vi "Keithley_IV Sweep.vi"() -> ()   [LabVIEW 2023]
uses:
  <instrlib>/Keithley 24XX/Public/Data/Read (Multiple Points).vi
  <vilib>/Utility/file.llb/Write Delimited Spreadsheet (DBL).vi
  <instrlib>/Keithley 24XX/Keithley 24XX.lvlib
  <vilib>/Analysis/NI_AALBase.lvlib
panel:
  in  "Current Range":i32(ring)=9 items=["mA"=3, "uA"=6, "nA"=9, "pA"=12]
  in  "path1 (folder + filename)":string="C:\\Users\\Carter Fox\\Documents\\probe data\\haolin\\"
  in  "Clear Plot":bool
  out "V-R":cluster{dbl[], dbl[]}(graph)={array[210 elements], [-5206154.0, -5436176.5, -5739949.7, -5522194.0, -5591894.0, -5776459.2, -5867751.5, -6153851.6, -6313039.5, -6546061.5, -6597968.0, -6737600.2, -6698442.5, -7003709.2, -7214062.5, -7227454.5, -7272324.7, -7315603.9, -8180765.4, -8370442.8, -8414466.4, -8558549.3, -8623235.6, -8485305.5, -8755154.4, -8913668.4, -8903585.8, -9356989.8, -9704273.0, -9888072.0, -9952694.2, -9462271.8, -9546720.8, -9151506.4, -9245727.0, -9130111.6, -8978078.6, -8980554.6, -8489626.5, -8766153.2, -8319403.2, -8056017.5, -8056376.9, -8148951.2, -8290770.6, -8061892.8, -8432694.3, -7918641.3, -7639503.0, -7371750.2, -7094581.9, -7089260.7, -6911397.3, -6586929.4, -6559722.9, -6559116.8, -6675187.5, -6447627.2, -6482316.2, -6441410.0, -6243156.7, -6007642.8, -5846703.5, -5641418.7, -5340011.0, -5222064.5, -5127084.4, -4771776.9, -4726834.2, -4488893.0, -4468031.1, -4344945.0, -4048716.15, -3995032.65, -3752934.4, -3515571.6, -3463041.0, -3307454.35, -3134452.0, -2865820.95, -2547093.35, -2451008.65, -2457232.75, -2264473.6, -2175654.9, -2075257.2, -1909759.55, -1690629.675, -1579277.55, -1439608.375, -1373833.05, -1280688.85, -1160609.625, -1028561.1, -853697.775, -738975.9375, -562712.525, -421306.975, -280443.56875, -143034.9875, 63.17793960571289, 142192.96875, 291373.54375, 450531.90625, 621629.55, 768361.2125, 936739.7125, 1078183.425, 1179651.7, 1308632.225, 1450103.325, 1578941.4, 1695594.975, 1815470.625, 2031218.15, 2205003.75, 2328910.65, 2527442.05, 2713821.7, 2773816.05, 2956326.5, 3094152.75, 3352913.7, 3405746.95, 3650903.3, 3816338.6, 3902421.4, 4254766.2, 4020501.7, 4199413.25, 4104189.3, 4316808.8, 4500217.9, 4625444.2, 4743101.6, 4847240.1, 4922873.9, 4963421.7, 5222360.7, 5435161.8, 5710479.7, 5953065.3, 5751540.2, 6185232.5, 6362707.2, 6258723.7, 6472245.0, 6749964.3, 6819459.9, 7089945.2, 7093988.2, 7265070.4, 7419388.4, 7450760.6, 7840890.3, 8010362.7, 8154184.9, 8595993.2, 8615776.8, 8657309.2, 8661124.2, 9076304.6, 8945453.0, 8963302.6, 9164656.4, 8956432.8, 9417630.4, 9845593.0, 9819956.8, 9964719.4, 9728544.4, 9516818.0, 9817531.6, 9995574.4, 9686989.6, 9619119.0, 9093431.0, 9016631.4, 9295223.0, 9272582.4, 9244173.2, 9498271.4, 8724864.2, 8299565.0, 8137673.6, 8124835.6, 8086662.6, 8106061.7, 7453452.1, 7138170.5, 6848874.7, 6885388.3, 6666333.2, 6471642.2, 6353635.0, 5981459.0, 5628015.5, 5593445.0, 5523823.4, 5316410.3, 5433694.8, 5403524.7, 5133651.1, 4923655.6, 4705024.7, 4949501.6, 4856533.7, 4489112.1, 4293774.4, 4293774.4]}
  out "I-R":cluster{dbl[], dbl[]}(graph)={array[210 elements], [-5206154.0, -5436176.5, -5739949.7, -5522194.0, -5591894.0, -5776459.2, -5867751.5, -6153851.6, -6313039.5, -6546061.5, -6597968.0, -6737600.2, -6698442.5, -7003709.2, -7214062.5, -7227454.5, -7272324.7, -7315603.9, -8180765.4, -8370442.8, -8414466.4, -8558549.3, -8623235.6, -8485305.5, -8755154.4, -8913668.4, -8903585.8, -9356989.8, -9704273.0, -9888072.0, -9952694.2, -9462271.8, -9546720.8, -9151506.4, -9245727.0, -9130111.6, -8978078.6, -8980554.6, -8489626.5, -8766153.2, -8319403.2, -8056017.5, -8056376.9, -8148951.2, -8290770.6, -8061892.8, -8432694.3, -7918641.3, -7639503.0, -7371750.2, -7094581.9, -7089260.7, -6911397.3, -6586929.4, -6559722.9, -6559116.8, -6675187.5, -6447627.2, -6482316.2, -6441410.0, -6243156.7, -6007642.8, -5846703.5, -5641418.7, -5340011.0, -5222064.5, -5127084.4, -4771776.9, -4726834.2, -4488893.0, -4468031.1, -4344945.0, -4048716.15, -3995032.65, -3752934.4, -3515571.6, -3463041.0, -3307454.35, -3134452.0, -2865820.95, -2547093.35, -2451008.65, -2457232.75, -2264473.6, -2175654.9, -2075257.2, -1909759.55, -1690629.675, -1579277.55, -1439608.375, -1373833.05, -1280688.85, -1160609.625, -1028561.1, -853697.775, -738975.9375, -562712.525, -421306.975, -280443.56875, -143034.9875, 63.17793960571289, 142192.96875, 291373.54375, 450531.90625, 621629.55, 768361.2125, 936739.7125, 1078183.425, 1179651.7, 1308632.225, 1450103.325, 1578941.4, 1695594.975, 1815470.625, 2031218.15, 2205003.75, 2328910.65, 2527442.05, 2713821.7, 2773816.05, 2956326.5, 3094152.75, 3352913.7, 3405746.95, 3650903.3, 3816338.6, 3902421.4, 4254766.2, 4020501.7, 4199413.25, 4104189.3, 4316808.8, 4500217.9, 4625444.2, 4743101.6, 4847240.1, 4922873.9, 4963421.7, 5222360.7, 5435161.8, 5710479.7, 5953065.3, 5751540.2, 6185232.5, 6362707.2, 6258723.7, 6472245.0, 6749964.3, 6819459.9, 7089945.2, 7093988.2, 7265070.4, 7419388.4, 7450760.6, 7840890.3, 8010362.7, 8154184.9, 8595993.2, 8615776.8, 8657309.2, 8661124.2, 9076304.6, 8945453.0, 8963302.6, 9164656.4, 8956432.8, 9417630.4, 9845593.0, 9819956.8, 9964719.4, 9728544.4, 9516818.0, 9817531.6, 9995574.4, 9686989.6, 9619119.0, 9093431.0, 9016631.4, 9295223.0, 9272582.4, 9244173.2, 9498271.4, 8724864.2, 8299565.0, 8137673.6, 8124835.6, 8086662.6, 8106061.7, 7453452.1, 7138170.5, 6848874.7, 6885388.3, 6666333.2, 6471642.2, 6353635.0, 5981459.0, 5628015.5, 5593445.0, 5523823.4, 5316410.3, 5433694.8, 5403524.7, 5133651.1, 4923655.6, 4705024.7, 4949501.6, 4856533.7, 4489112.1, 4293774.4, 4293774.4]}
  out "I-V":cluster{dbl[], dbl[]}(graph)
  out "V-I":cluster{dbl[], dbl[]}(graph)
  in  "Sample Count":i32=5
  out "R error":dbl=149486.27445061636 format="%0.2f"
  out "R":dbl=-5206154.0 format="%0.2f"
  out "I error":dbl=22.839692677696984 format="%0.2f"
  out "I":dbl=769.2151598348573 format="%0.2f"
  out "V error":dbl=2.768120817890166e-06 format="%0.2f"
  out "V":dbl=-4.001921558380127 format="%0.2f"
  in  "Source Mode  (0: Voltage)":u16(ring) items=["Voltage", "Current"]
  in  "Compliance  Level":dbl=0.1
  in  "milliseconds to wait":u32=10
  in  "Serial Configuration":T1={"Baud Rate"=9600, "Parity"=0, "Data Bits"=8, "Stop Bits"=10, "Flow Control"=0} {"Flow Control" items=["None", "XON/XOFF", "RTS/CTS", "XON/XOFF & RTS/CTS", "DTR/DSR", "XON/XOFF & DTR/DSR"]; "Stop Bits" items=["1.0"=10, "1.5"=15, "2.0"=20]; "Data Bits" items=["7"=7, "8"=8]; "Parity" items=["None", "Odd", "Even", "Mark", "Space"]; "Baud Rate" items=["300"=300, "600"=600, "1200"=1200, "2400"=2400, "4800"=4800, "9600"=9600, "19200"=19200]}
  in  "VISA resource name":refnum<visa-resource-name>="GPIB0::16::INSTR"
  in  "End Point 1 (V/A)":dbl=7.0
  in  "Region 2":bool
  in  "End Point 2 (V/A)":dbl=7.0
  in  "Step 2 (mV/mA)":dbl=100.0
  in  "Step 1 (mV/mA)":dbl=100.0
  in  "Starting Point (V/A)":dbl
  in  "Single/Double":i32=2 min=1 max=2 step=1
  out "Backward":bool
  out "Forward":bool=TRUE
  out "Region 1 steps":dbl=70.0
  out "Region 2  steps":dbl
  out "loop run":i32=1
  in  "loop #":i32=2
  in  "Save data or not":bool=TRUE
  out "SD voltage":dbl=-3.9 format="%#_13g"
  # "Keithley Setting"
  # "Sweeping Setting"
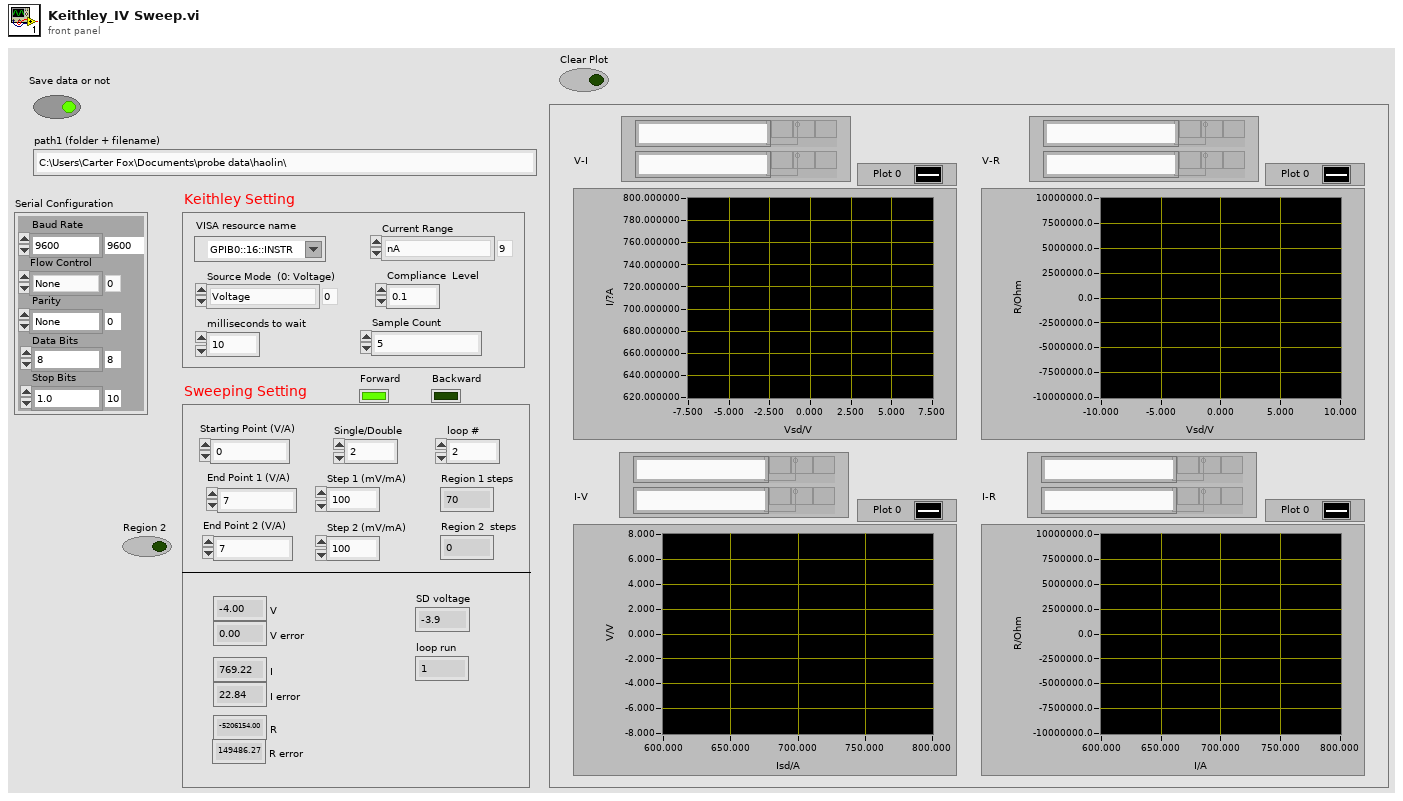
[diagram p1: front panel]
types:
  T1 = cluster{"Baud Rate":u32, "Parity":u16, "Data Bits":u16, "Stop Bits":u16, "Flow Control":u16}
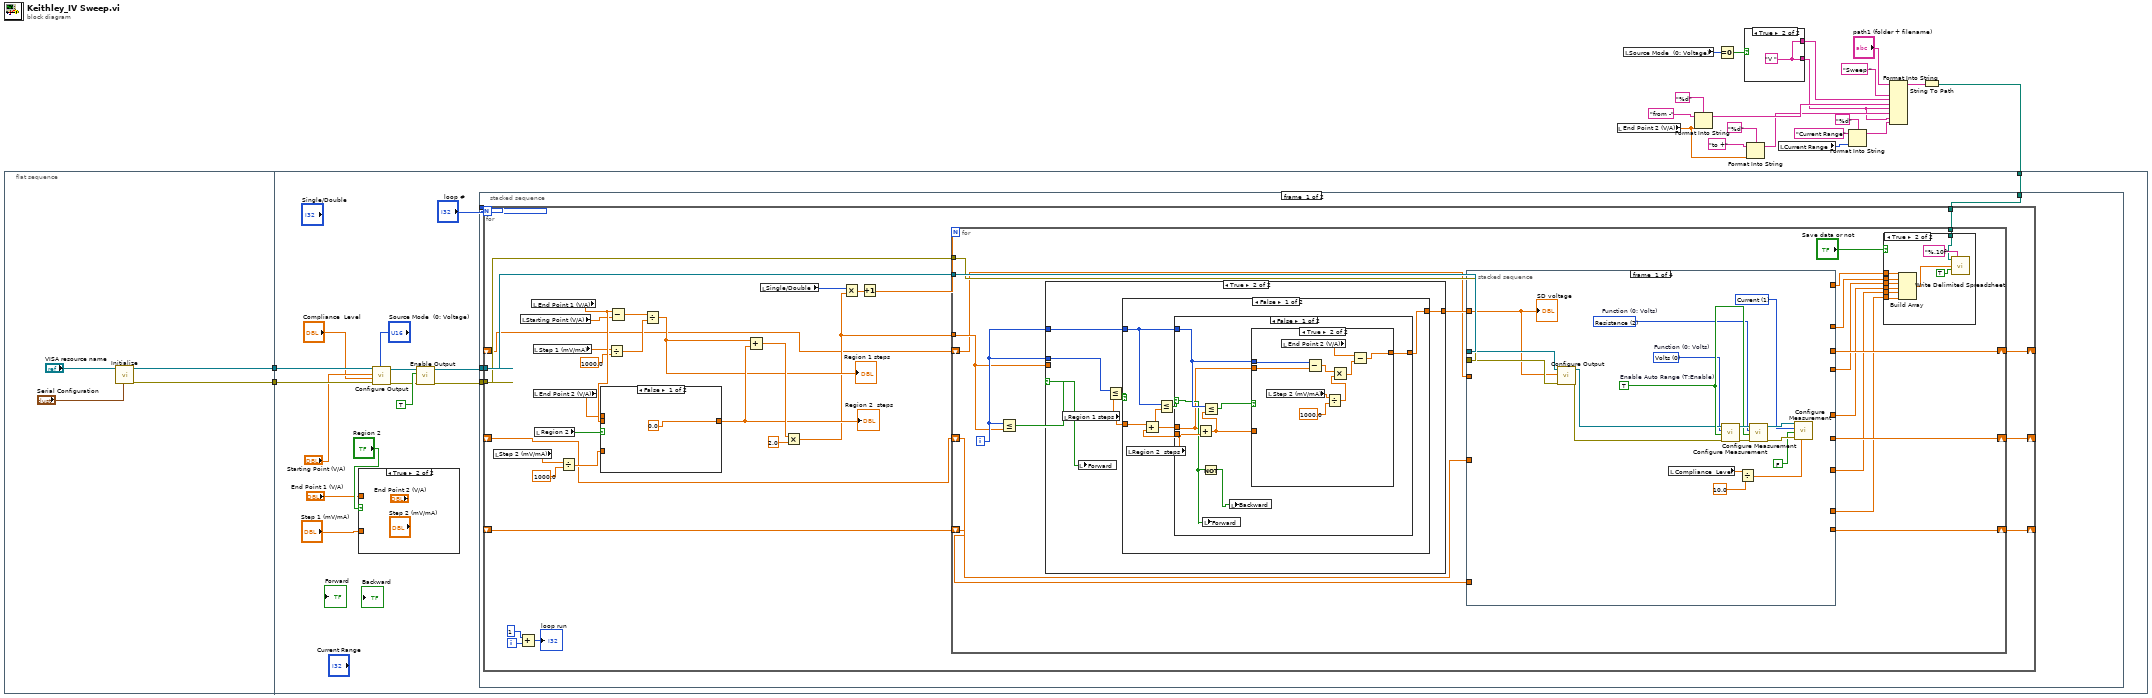
[diagram p0: block diagram]
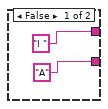
[diagram p2: hidden frame]
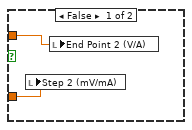
[diagram p3: hidden frame]
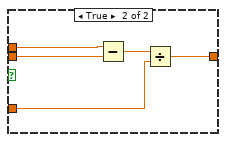
[diagram p4: hidden frame]
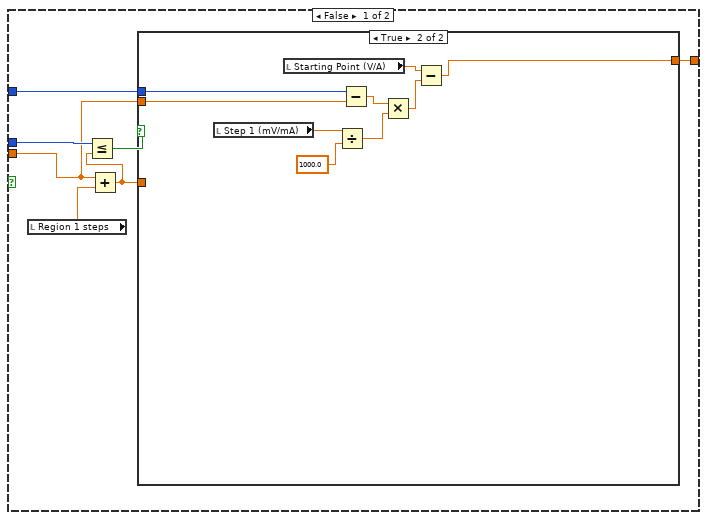
[diagram p5: hidden frame]
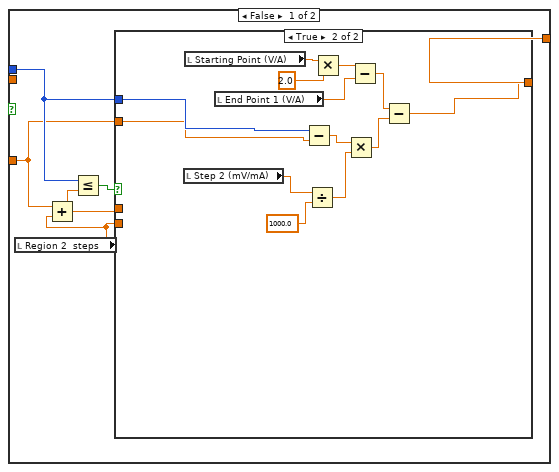
[diagram p6: hidden frame]
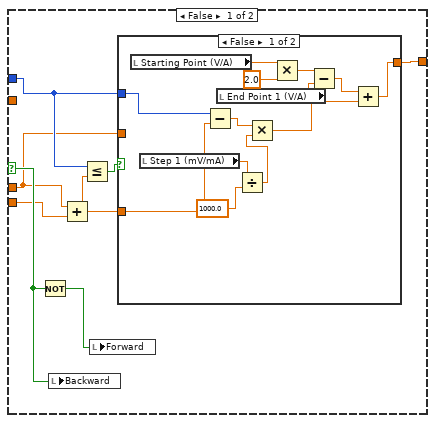
[diagram p7: hidden frame]
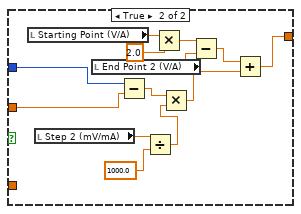
[diagram p8: hidden frame]
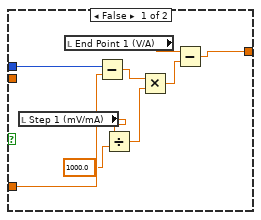
[diagram p9: hidden frame]
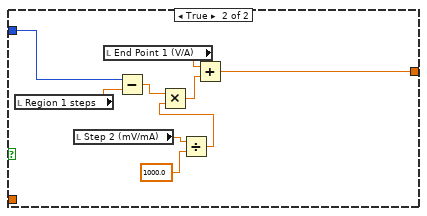
[diagram p10: hidden frame]
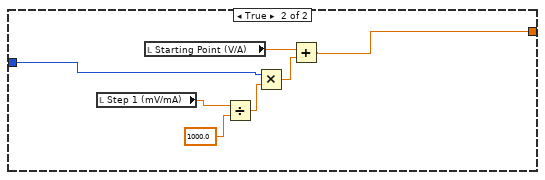
[diagram p11: hidden frame]
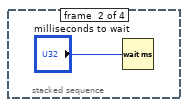
[diagram p13: hidden frame]
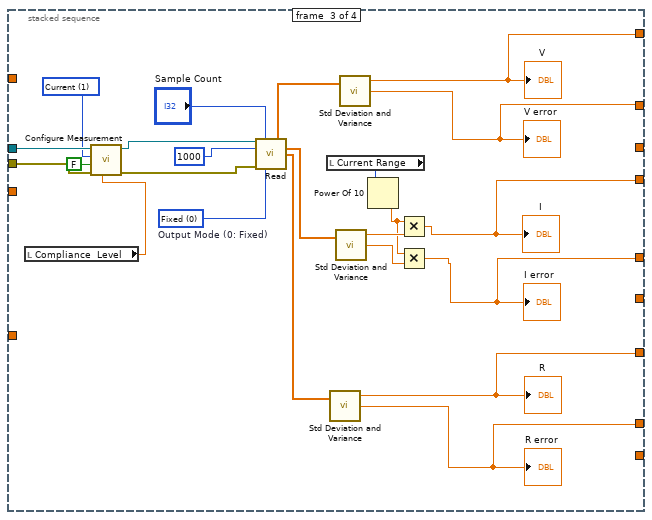
[diagram p14: hidden frame]
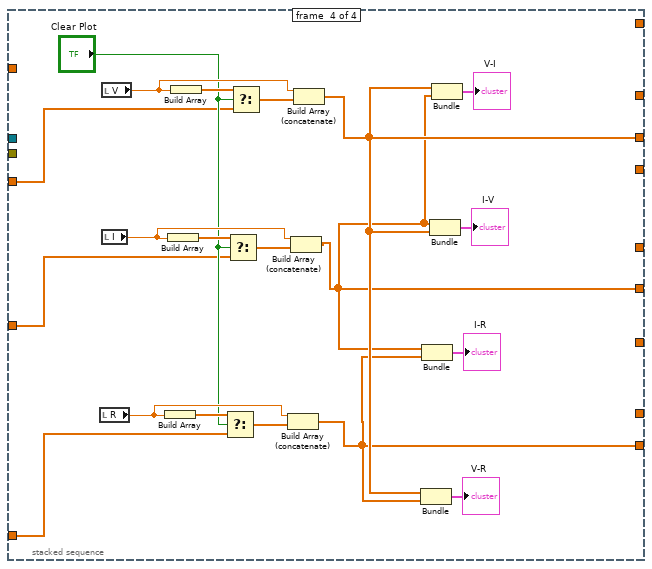
[diagram p15: hidden frame]
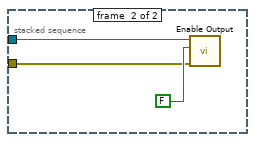
[diagram p16: hidden frame]
diagram:
  n1 = flat-sequence {
    tunnel: [w23] -> w21
    tunnel: [w22] -> w20
    tunnel: w21 -> [w33]
    tunnel: w20 -> [w32]
    tunnel: w17 -> [w26]
    frame #0 {
      n2 = call <instrlib>:"Initialize.vi"("Serial Configuration"="Serial Configuration", "VISA resource name"="VISA resource name") -> ("error out"=w22:errorcluster, "VISA resource name out"=w23:refnum<visa-resource-name>)  [unwired: 8 in]
    }
    frame #1 {
      n3 = case shown="True" "Region 2" {
        tunnel: "End Point 1 (V/A)" -> [w42 _]
        tunnel: "Step 1 (mV/mA)" -> [w41 _]
        frame False {
          n4 = local write "Step 2 (mV/mA)"(w41) -> ()
          n5 = local write "End Point 2 (V/A)"(w42) -> ()
        }
        frame True {
        }
      }
      n6 = call <instrlib>:"Configure Output.vi"("Source Mode  (0: Voltage)"="Source Mode  (0: Voltage)", "error in (no error)"=w32, "Compliance  Level (0.1)"="Compliance  Level", "Output Level (0)"="Starting Point (V/A)", "VISA resource name"=w33) -> ("error out"=w35:errorcluster, "VISA resource name out"=w34:refnum<visa-resource-name>)  [unwired: 5 in]
      n7 = call <instrlib>:"Enable Output.vi"("error in (no error)"=w35, "Enable Output (T: Enable)"=TRUE, "VISA resource name"=w34) -> ("error out"=w30:errorcluster, "VISA resource name out"=w31:refnum<visa-resource-name>)  [unwired: 7 in]
      n8 = stacked-sequence {
        tunnel: "loop #" -> [w46 _]
        tunnel: w31 -> [w45 w299]
        tunnel: w30 -> [w44 w298]
        tunnel: w26 -> [w43 _]
        frame #0 {
          n9 = for {
            N: w46 -> [_]
            tunnel: w45 -> [w77]
            tunnel: w44 -> [w60]
            shift-right: [w53] -> _
            shift-left: _ -> [w52]
            shift-right: [w51] -> _
            shift-left: _ -> [w50]
            shift-right: [w49] -> _
            shift-left: _ -> [w48]
            tunnel: w43 -> [w47]
            i -> [w75]
            n10 = local read "Step 2 (mV/mA)"() -> (w56:dbl)
            n11 = Add(x=1, y=w75) -> (x+y=→"loop run":i32)
            n12 = local read "Starting Point (V/A)"() -> (w70:dbl)
            n13 = local read "End Point 1 (V/A)"() -> (w72:dbl)
            n14 = local read "Step 1 (mV/mA)"() -> (w57:dbl)
            n15 = local read "End Point 2 (V/A)"() -> (w71:dbl)
            n16 = local read "Region 2"() -> (w67:bool)
            n17 = Divide(x=w56, y=1000.0) -> (x/y=w54:dbl)
            n18 = case shown="False" w67 {
              tunnel: w72 -> [_ w82]
              tunnel: [0.0 w81] -> w69
              tunnel: w54 -> [_ w80]
              tunnel: w71 -> [_ w79]
              frame False {
              }
              frame True {
                n19 = Subtract(x=w79, y=w82) -> (x-y=w83:dbl)
                n20 = Divide(x=w83, y=w80) -> (x/y=w81:dbl)
              }
            }
            "Region 2  steps" <- w69
            n21 = Divide(x=w57, y=1000.0) -> (x/y=w59:dbl)
            n22 = Subtract(x=w72, y=w70) -> (x-y=w64:dbl)
            n23 = Divide(x=w64, y=w59) -> (x/y=w68:dbl)
            "Region 1 steps" <- w68
            n24 = Add(x=w68, y=w69) -> (x+y=w73:dbl)
            n25 = local read "Single/Double"() -> (w66:i32)
            n26 = Multiply(x=w73, y=2.0) -> (x*y=w61:dbl)
            n27 = Multiply(x=w66, y=w61) -> (x*y=w65:dbl)
            n28 = Increment(x=w65) -> (x+1=w62:dbl)
            n29 = for {
              N: w62 -> [_]
              tunnel: w77 -> [w103]
              tunnel: w61 -> [w99]
              tunnel: w60 -> [w97]
              shift-right: [w96] -> w53
              shift-left: w52 -> [w95]
              shift-right: [w94] -> w51
              shift-left: w50 -> [w93]
              shift-right: [w92] -> w49
              shift-left: w48 -> [w91]
              tunnel: w47 -> [w84]
              i -> [w100]
              n30 = Less Or Equal?(x=w100, y=w99) -> (x <= y?=w101:bool)
              n31 = case shown="True" w101 {
                selector: w101 -> [_ w174]
                tunnel: w100 -> [w110 w178]
                tunnel: [w106 w177] -> w98
                tunnel: w100 -> [w109 w176]
                tunnel: w99 -> [w105 _]
                frame False {
                  n32 = local read "Region 1 steps"() -> (w107:dbl)
                  n33 = Add(x=w105, y=w107) -> (x+y=w104:dbl)
                  n34 = Less Or Equal?(x=w109, y=w104) -> (x <= y?=w108:bool)
                  n35 = case shown="True" w108 {
                    tunnel: w110 -> [w114 w172]
                    tunnel: [w115 w169] -> w106
                    tunnel: w105 -> [_ w168]
                    tunnel: w104 -> [w113 _]
                    frame False {
                      n36 = local read "Region 2  steps"() -> (w111:dbl)
                      n37 = Add(x=w113, y=w111) -> (x+y=w112:dbl)
                      n38 = Less Or Equal?(x=w114, y=w112) -> (x <= y?=w116:bool)
                      n39 = case shown="True" w116 {
                        selector: w116 -> [w123 _]
                        tunnel: [w124 w163] -> w115
                        tunnel: w114 -> [w119 w162]
                        tunnel: w113 -> [_ w161]
                        tunnel: w112 -> [w118 _]
                        tunnel: w111 -> [w120 _]
                        frame False {
                          n40 = Not(x=w123) -> (.not. x?=w122:bool)
                          n41 = local write "Backward"(w123) -> ()
                          n42 = Add(x=w118, y=w120) -> (x+y=w117:dbl)
                          n43 = Less Or Equal?(x=w119, y=w117) -> (x <= y?=w121:bool)
                          n44 = local write "Forward"(w122) -> ()
                          n45 = case shown="False" w121 {
                            tunnel: [w134 w149] -> w124
                            tunnel: w119 -> [w133 w148]
                            tunnel: w118 -> [_ w147]
                            tunnel: w117 -> [w132 _]
                            frame False {
                              n46 = local read "Starting Point (V/A)"() -> (w130:dbl)
                              n47 = local read "Step 1 (mV/mA)"() -> (w126:dbl)
                              n48 = Subtract(x=w133, y=w132) -> (x-y=w131:dbl)
                              n49 = local read "End Point 1 (V/A)"() -> (w128:dbl)
                              n50 = Divide(x=w126, y=1000.0) -> (x/y=w125:dbl)
                              n51 = Multiply(x=w131, y=w125) -> (x*y=w137:dbl)
                              n52 = Multiply(x=w130, y=2.0) -> (x*y=w136:dbl)
                              n53 = Subtract(x=w136, y=w128) -> (x-y=w135:dbl)
                              n54 = Add(x=w135, y=w137) -> (x+y=w134:dbl)
                            }
                            frame True {
                              n55 = local read "Starting Point (V/A)"() -> (w144:dbl)
                              n56 = local read "Step 2 (mV/mA)"() -> (w139:dbl)
                              n57 = local read "End Point 2 (V/A)"() -> (w141:dbl)
                              n58 = Subtract(x=w148, y=w147) -> (x-y=w142:dbl)
                              n59 = Divide(x=w139, y=1000.0) -> (x/y=w138:dbl)
                              n60 = Multiply(x=w144, y=2.0) -> (x*y=w146:dbl)
                              n61 = Multiply(x=w142, y=w138) -> (x*y=w150:dbl)
                              n62 = Subtract(x=w146, y=w141) -> (x-y=w145:dbl)
                              n63 = Add(x=w145, y=w150) -> (x+y=w149:dbl)
                            }
                          }
                        }
                        frame True {
                          n64 = local read "Step 2 (mV/mA)"() -> (w152:dbl)
                          n65 = local read "Starting Point (V/A)"() -> (w157:dbl)
                          n66 = local read "End Point 1 (V/A)"() -> (w155:dbl)
                          n67 = Subtract(x=w162, y=w161) -> (x-y=w159:dbl)
                          n68 = Divide(x=w152, y=1000.0) -> (x/y=w151:dbl)
                          n69 = Multiply(x=w157, y=2.0) -> (x*y=w158:dbl)
                          n70 = Multiply(x=w159, y=w151) -> (x*y=w160:dbl)
                          n71 = Subtract(x=w158, y=w155) -> (x-y=w154:dbl)
                          n72 = Subtract(x=w154, y=w160) -> (x-y=w163:dbl)
                        }
                      }
                    }
                    frame True {
                      n73 = local read "Step 1 (mV/mA)"() -> (w165:dbl)
                      n74 = local read "Starting Point (V/A)"() -> (w170:dbl)
                      n75 = Divide(x=w165, y=1000.0) -> (x/y=w164:dbl)
                      n76 = Subtract(x=w172, y=w168) -> (x-y=w167:dbl)
                      n77 = Multiply(x=w167, y=w164) -> (x*y=w171:dbl)
                      n78 = Subtract(x=w170, y=w171) -> (x-y=w169:dbl)
                    }
                  }
                }
                frame True {
                  n79 = local read "Region 1 steps"() -> (w173:dbl)
                  n80 = local write "Forward"(w174) -> ()
                  n81 = Less Or Equal?(x=w176, y=w173) -> (x <= y?=w175:bool)
                  n82 = case shown="False" w175 {
                    tunnel: w178 -> [w182 w224]
                    tunnel: [w181 w225] -> w177
                    tunnel: w173 -> [w183 _]
                    frame False {
                      n83 = local read "Region 2  steps"() -> (w179:dbl)
                      n84 = Add(x=w183, y=w179) -> (x+y=w180:dbl)
                      n85 = Less Or Equal?(x=w182, y=w180) -> (x <= y?=w184:bool)
                      n86 = case shown="False" w184 {
                        selector: w184 -> [w188 _]
                        tunnel: w182 -> [w191 w217]
                        tunnel: [w192 w214] -> w181
                        tunnel: w180 -> [w186 _]
                        tunnel: w179 -> [w190 _]
                        frame False {
                          n87 = Add(x=w186, y=w190) -> (x+y=w185:dbl)
                          n88 = Not(x=w188) -> (.not. x?=w187:bool)
                          n89 = Less Or Equal?(x=w191, y=w185) -> (x <= y?=w189:bool)
                          n90 = local write "Forward"(w188) -> ()
                          n91 = local write "Backward"(w187) -> ()
                          n92 = case shown="True" w189 {
                            tunnel: w191 -> [w198 w207]
                            tunnel: [w196 w206] -> w192
                            tunnel: w186 -> [_ w205]
                            tunnel: w185 -> [w197 _]
                            frame False {
                              n93 = local read "Step 1 (mV/mA)"() -> (w194:dbl)
                              n94 = local read "End Point 1 (V/A)"() -> (w199:dbl)
                              n95 = Subtract(x=w198, y=w197) -> (x-y=w201:dbl)
                              n96 = Divide(x=w194, y=1000.0) -> (x/y=w193:dbl)
                              n97 = Multiply(x=w201, y=w193) -> (x*y=w200:dbl)
                              n98 = Subtract(x=w199, y=w200) -> (x-y=w196:dbl)
                            }
                            frame True {
                              n99 = local read "Step 2 (mV/mA)"() -> (w203:dbl)
                              n100 = local read "End Point 2 (V/A)"() -> (w208:dbl)
                              n101 = Subtract(x=w207, y=w205) -> (x-y=w210:dbl)
                              n102 = Divide(x=w203, y=1000.0) -> (x/y=w202:dbl)
                              n103 = Multiply(x=w210, y=w202) -> (x*y=w209:dbl)
                              n104 = Subtract(x=w208, y=w209) -> (x-y=w206:dbl)
                            }
                          }
                        }
                        frame True {
                          n105 = local read "Region 1 steps"() -> (w216:dbl)
                          n106 = local read "Step 2 (mV/mA)"() -> (w213:dbl)
                          n107 = local read "End Point 1 (V/A)"() -> (w218:dbl)
                          n108 = Subtract(x=w217, y=w216) -> (x-y=w215:dbl)
                          n109 = Divide(x=w213, y=1000.0) -> (x/y=w211:dbl)
                          n110 = Multiply(x=w215, y=w211) -> (x*y=w219:dbl)
                          n111 = Add(x=w218, y=w219) -> (x+y=w214:dbl)
                        }
                      }
                    }
                    frame True {
                      n112 = local read "Step 1 (mV/mA)"() -> (w221:dbl)
                      n113 = local read "Starting Point (V/A)"() -> (w223:dbl)
                      n114 = Divide(x=w221, y=1000.0) -> (x/y=w220:dbl)
                      n115 = Multiply(x=w224, y=w220) -> (x*y=w226:dbl)
                      n116 = Add(x=w223, y=w226) -> (x+y=w225:dbl)
                    }
                  }
                }
              }
              n117 = stacked-sequence {
                tunnel: w103 -> [w252 _ w267 _]
                tunnel: w97 -> [w253 _ w266 _]
                tunnel: w98 -> [w251 _ _ _]
                tunnel: [_ _ _ w283] -> w96
                tunnel: w95 -> [_ _ _ w278]
                tunnel: [_ _ _ w282] -> w94
                tunnel: w93 -> [_ _ _ w279]
                tunnel: [_ _ _ w281] -> w92
                tunnel: w91 -> [_ _ _ w280]
                tunnel: [_ _ w271 _] -> w90
                tunnel: [_ _ w270 _] -> w89
                tunnel: [_ _ w258 _] -> w88
                tunnel: [_ _ w255 _] -> w87
                tunnel: [_ _ w269 _] -> w86
                tunnel: [_ _ w268 _] -> w85
                frame #0 {
                  w245 = u16 1 items=["Volts", "Current", "Resistance"] ("Function (0: Volts)")
                  w246 = TRUE  # Enable Auto Range (T:Enable)
                  w244 = u16 2 items=["Volts", "Current", "Resistance"]  # Function (0: Volts)
                  w241 = u16 0 items=["Volts", "Current", "Resistance"]  # Function (0: Volts)
                  n118 = call <instrlib>:"Configure Output.vi"("error in (no error)"=w253, "Output Level (0)"=w251, "VISA resource name"=w252) -> ("error out"=w242:errorcluster, "VISA resource name out"=w243:refnum<visa-resource-name>)  [unwired: 7 in]
                  n119 = local read "Compliance  Level"() -> (w239:dbl)
                  n120 = call <instrlib>:"Configure Measurement.vi"("error in (no error)"=w242, "Enable Auto Range (T:Enable)"=w246, "Function (0: Volts)"=w241, "VISA resource name"=w243) -> ("error out"=w247:errorcluster, "VISA resource name out"=w248:refnum<visa-resource-name>)  [unwired: 6 in]
                  n121 = Divide(x=w239, y=10.0) -> (x/y=w237:dbl)
                  n122 = call <instrlib>:"Configure Measurement.vi"("error in (no error)"=w247, "Enable Auto Range (T:Enable)"=w246, "Function (0: Volts)"=w244, "VISA resource name"=w248) -> ("error out"=w250:errorcluster, "VISA resource name out"=w249:refnum<visa-resource-name>)  [unwired: 6 in]
                  n123 = call <instrlib>:"Configure Measurement.vi"("Manual Range (1.0)"=w237, "error in (no error)"=w250, "Enable Auto Range (T:Enable)"=FALSE, "Function (0: Volts)"=w245, "VISA resource name"=w249) -> ()  [unwired: 5 in, 2 out]
                  "SD voltage" <- w251
                }
                frame #1 {
                  n124 = Wait (ms)(milliseconds to wait="milliseconds to wait") -> ()  [unwired: 1 out]
                }
                frame #2 {
                  w263 = u16 1 items=["Volts", "Current", "Resistance"] ("Function (0: Volts)")
                  w276 = u16 0 items=["Fixed", "Sweep", "List"]  # Output Mode (0: Fixed)
                  n125 = local read "Compliance  Level"() -> (w261:dbl)
                  n126 = call <instrlib>:"Configure Measurement.vi"("Manual Range (1.0)"=w261, "error in (no error)"=w266, "Enable Auto Range (T:Enable)"=FALSE, "Function (0: Volts)"=w263, "VISA resource name"=w267) -> ("error out"=w265:errorcluster, "VISA resource name out"=w264:refnum<visa-resource-name>)  [unwired: 5 in]
                  n127 = call-poly <instrlib>:"Read.vi"("VISA resource name"=w264, "Sample Count (1)"="Sample Count", "Timeout (10000 ms)"=1000, "error in (no error)"=w265, "Output Mode (0: Fixed)"=w276) -> ("Voltage"=w274:sgl[], "Current"=w275:sgl[], "Resistance"=w273:sgl[])  [unwired: 4 in, 4 out]
                  n128 = local read "Current Range"() -> (w260:i32)
                  n129 = call <vilib>:"Std Deviation and Variance.vi"("X"=w273) -> ("mean"=w269:dbl, "standard deviation"=w268:dbl)  [unwired: 1 in, 1 out]
                  "R" <- w269
                  "R error" <- w268
                  n130 = call <vilib>:"Std Deviation and Variance.vi"("X"=w275) -> ("mean"=w259:dbl, "standard deviation"=w257:dbl)  [unwired: 1 in, 1 out]
                  n131 = call <vilib>:"Std Deviation and Variance.vi"("X"=w274) -> ("mean"=w271:dbl, "standard deviation"=w270:dbl)  [unwired: 1 in, 1 out]
                  "V" <- w271
                  "V error" <- w270
                  n132 = Power Of 10(x=w260) -> (10^x=w256:dbl)
                  n133 = Multiply(x=w256, y=w259) -> (x*y=w258:dbl)
                  "I" <- w258
                  n134 = Multiply(x=w256, y=w257) -> (x*y=w255:dbl)
                  "I error" <- w255
                }
                frame #3 {
                  n135 = local read "R"() -> (w285:dbl)
                  n136 = local read "V"() -> (w296:dbl)
                  n137 = local read "I"() -> (w286:dbl)
                  n138 = Build Array(w285) -> (w288:dbl[])
                  n139 = Build Array(w286) -> (w290:dbl[])
                  n140 = Build Array(w296) -> (w297:dbl[])
                  n141 = Select(t=w288, s="Clear Plot", f=w280) -> (s? t:f=w287:dbl[])
                  n142 = Select(t=w290, s="Clear Plot", f=w279) -> (s? t:f=w289:dbl[])
                  n143 = Select(t=w297, s="Clear Plot", f=w278) -> (s? t:f=w295:dbl[])
                  n144 = Build Array (concatenate)(w285, w287) -> (w281:dbl[])
                  n145 = Build Array (concatenate)(w286, w289) -> (w282:dbl[])
                  n146 = Build Array (concatenate)(w296, w295) -> (w283:dbl[])
                  n147 = Bundle(w283, w281) -> (→"V-R":cluster{dbl[], dbl[]})  [unwired: 1 in]
                  n148 = Bundle(w282, w281) -> (→"I-R":cluster{dbl[], dbl[]})  [unwired: 1 in]
                  n149 = Bundle(w282, w283) -> (→"I-V":cluster{dbl[], dbl[]})  [unwired: 1 in]
                  n150 = Bundle(w283, w282) -> (→"V-I":cluster{dbl[], dbl[]})  [unwired: 1 in]
                }
              }
              n151 = case shown="True" "Save data or not" {
                tunnel: w90 -> [_ w233]
                tunnel: w89 -> [_ w232]
                tunnel: w88 -> [_ w231]
                tunnel: w87 -> [_ w230]
                tunnel: w86 -> [_ w229]
                tunnel: w85 -> [_ w228]
                tunnel: w84 -> [_ w227]
                frame False {
                }
                frame True {
                  n152 = Build Array(w233, w232, w231, w230, w229, w228) -> (w236:dbl[])
                  n153 = call-poly <vilib>:"Write Delimited Spreadsheet.vi"("file path (dialog if empty)"=w227, "format (%.3f)"="%.10f", "1D data"=w236, "append to file? (new file:F)"=TRUE) -> ()  [unwired: 10 in, 2 out]
                }
              }
            }
          }
        }
        frame #1 {
          n154 = call <instrlib>:"Enable Output.vi"("error in (no error)"=w298, "Enable Output (T: Enable)"=FALSE, "VISA resource name"=w299) -> ()  [unwired: 7 in, 2 out]
        }
      }
    }
  }
  n155 = local read "End Point 2 (V/A)"() -> (w7:dbl)
  n156 = local read "Source Mode  (0: Voltage)"() -> (w16:u16)
  n157 = Format Into String(format string="%d", initial string="from -", w7) -> (resulting string=w10:string)  [unwired: 1 in, 1 out]
  n158 = Equal To 0?(x=w16) -> (x = 0?=w15:bool)
  n159 = case shown="True" w15 {
    tunnel: ["I " ("input 1") w303] -> w13
    tunnel: ["A" ("input 1") w303] -> w5
    frame False {
    }
    frame True {
      w303 = "V " ("input 1")
    }
  }
  n160 = Format Into String(format string="%d", initial string="to +", w7) -> (resulting string=w6:string)  [unwired: 1 in, 1 out]
  n161 = local read "Current Range"() -> (w4:i32)
  n162 = Format Into String(format string="%d", initial string="Current Range", w4) -> (resulting string=w2:string)  [unwired: 1 in, 1 out]
  n163 = Format Into String(initial string="path1 (folder + filename)", "Sweep " ("input 1"), w13, w10, w5, w6, w5, w2) -> (resulting string=w18:string)  [unwired: 2 in, 1 out]
  n164 = String To Path(string=w18) -> (path=w17:path)
